vi "MB Serial Init.vi"(4 "Timeout":u32=10000, 6 "Flow Control":u16(ring) items=["None", "XON/XOFF", "RTS/CTS", "XON/XOFF & RTS/CTS", "DTR/DSR", "XON/XOFF & DTR/DSR"], 7 "Mode":enum16{"RTU", "ASCII"}(ring), 8 "error in (no error)":errorcluster, 9 "Parity":u16(ring) items=["None", "Odd", "Even", "Mark", "Space"], 10 "Baud Rate":u32=9600, 11 "VISA resource name":refnum<visa-resource-name>) -> (0 "error out":errorcluster, 3 "VISA resource name out":refnum<visa-resource-name>)   [LabVIEW 2020, in "ModBus Serial Master.lvlib"]
doc: "Initializes the serial port specified by VISA resource name to the specified settings. Wire data to the VISA resource name input to determine the polymorphic instance to use or manually select the instance."
uses:
  ModBus Serial Master.lvlib
  Common.lvlib
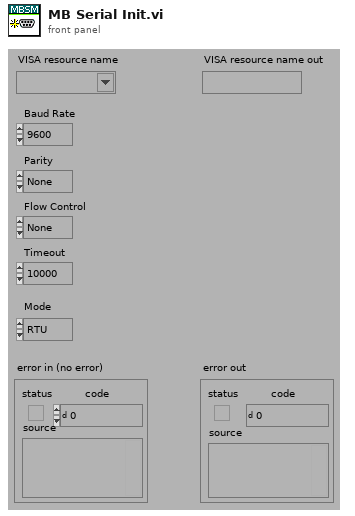
[diagram p1: front panel]
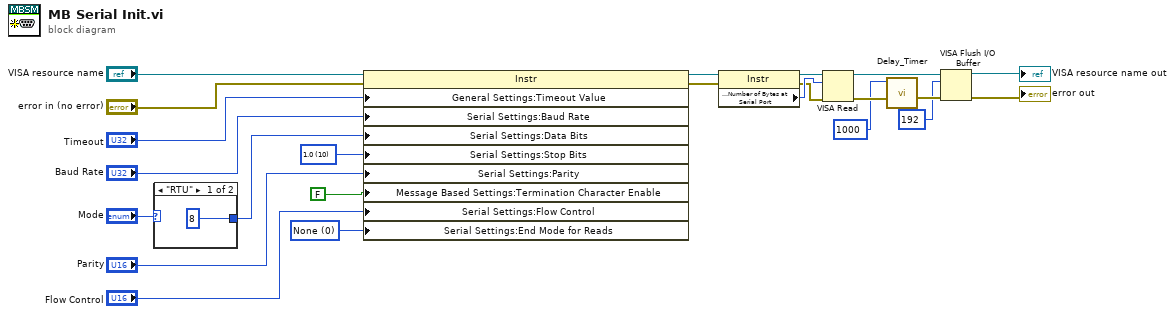
[diagram p0: block diagram]
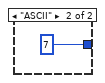
[diagram p2: hidden frame]
diagram:
  w20 = u16 0 items=["None", "LastBit", "TermChar"] ("Serial Settings:Serial End Mode for Reads")
  w22 = u16 10 items=["1.0"=10, "1.5"=15, "2.0"=20] ("Serial Settings:Serial Stop Bits")
  n1 = case shown="\"RTU\"" "Mode" {
    tunnel: [u16 8 ("data bits") u16 7 ("data bits")] -> w21
    frame "RTU" {
    }
    frame "ASCII" {
    }
  }
  n2 = property class="Instr"(reference="VISA resource name", error in="error in (no error)", "General Settings:Timeout Value"="Timeout", "Serial Settings:Baud Rate"="Baud Rate", "Serial Settings:Data Bits"=w21, "Serial Settings:Stop Bits"=w22, "Serial Settings:Parity"="Parity", "Message Based Settings:Termination Character Enable"=FALSE, "Serial Settings:Flow Control"="Flow Control", "Serial Settings:End Mode for Reads"=w20) -> (reference out=w11:refnum<visa-resource-name>, error out=w12:errorcluster)
  n3 = property class="Instr"(reference=w11, error in=w12) -> (reference out=w10:refnum<visa-resource-name>, error out=w8:errorcluster, "Serial Settings:Number of Bytes at Serial Port"=w9:u32)
  n4 = VISA Read(VISA resource name=w10, byte count=w9, error in (no error)=w8) -> (VISA resource name out=w4:refnum<visa-resource-name>, error out=w7:errorcluster)  [unwired: 2 out]
  n5 = call "Delay_Timer.vi"("error in (no error)"=w7, "Delay_Time(ms)"=u32 1000) -> ("error out"=w5:errorcluster)  [unwired: 9 in]
  n6 = VISA Flush I/O Buffer(VISA resource name=w4, mask (16)=u16 192, error in (no error)=w5) -> (VISA resource name out=→"VISA resource name out":refnum<visa-resource-name>, error out=→"error out":errorcluster)
